vi "VMI_save_IF32_format.vi"(3 "Image Array":i16[][](array[numeric]), 4 "Image Info":T2={"X size"=782.0, "Y size"=582.0, "Centroiding"=1.0}, 5 "Header Cluster":T1) -> (2 "File String":string)   [LabVIEW 2018]
uses:
  Type defs/Image_info.ctl
  Type defs/Header_infor_IF32.ctl
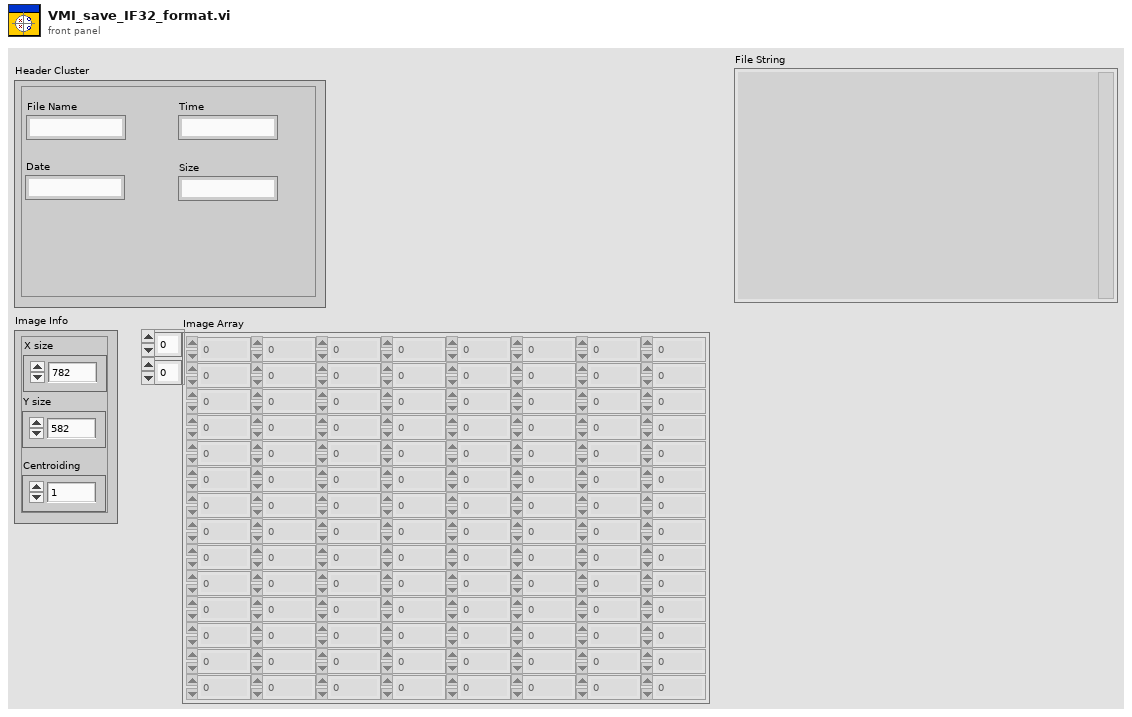
[diagram p1: front panel]
types:
  T1 = typedef "Header_infor_IF32.ctl" = cluster{"File Name":string, "Time":string, "Date":string, "Size":string}
  T2 = typedef "Image_info.ctl" = cluster{"X size":dbl, "Y size":dbl, "Centroiding":dbl}
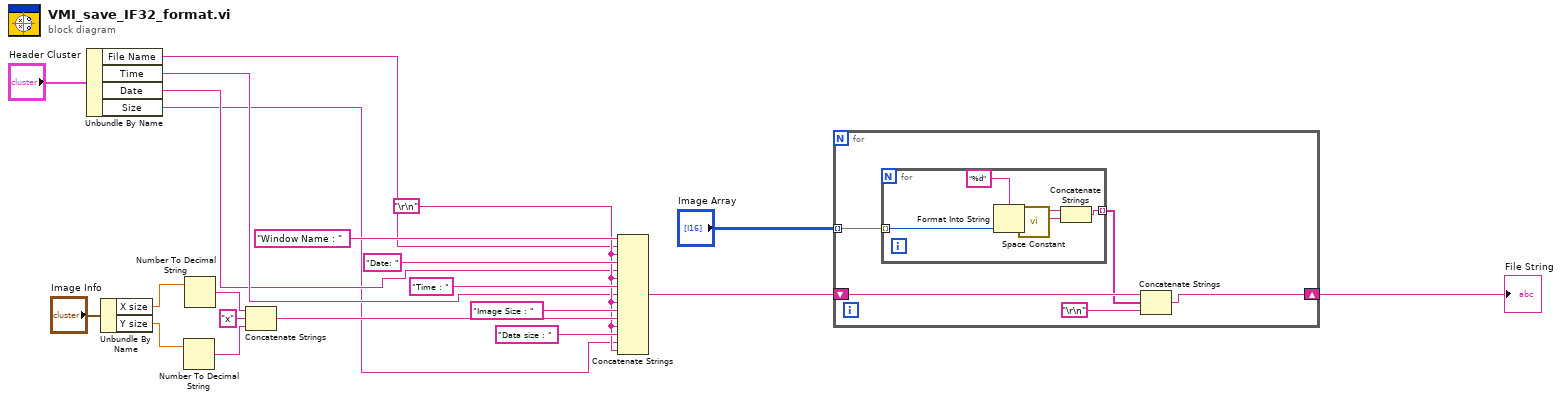
[diagram p0: block diagram]
diagram:
  w8 = "\r\n"
  n1 = Unbundle By Name("Header Cluster") -> ("File Name"=w4:string, "Time"=w3:string, "Date"=w2:string, "Size"=w1:string)
  n2 = Unbundle By Name("Image Info") -> ("X size"=w17:dbl, "Y size"=w16:dbl)
  n3 = Number To Decimal String(number=w16) -> (decimal integer string=w15:string)  [unwired: 1 in]
  n4 = Number To Decimal String(number=w17) -> (decimal integer string=w14:string)  [unwired: 1 in]
  n5 = Concatenate Strings(w14, "x" ("string"), w15) -> (w12:string)
  n6 = Concatenate Strings("Window Name : " ("string"), w4, w8, "Date: " ("string"), w2, w8, "Time : " ("string"), w3, w8, "Image Size : " ("string"), w12, w8, "Data size : " ("string"), w1, w8) -> (w7:string)
  n7 = for {
    tunnel: "Image Array" -> [w26] mode=indexing
    shift-right: [w22] -> w6
    shift-left: w7 -> [w25]
    n8 = for {
      tunnel: w26 -> [w31] mode=indexing
      tunnel: [w28] -> w24 mode=indexing
      n9 = Format Into String(format string="%d", w31) -> (resulting string=w30:string)  [unwired: 2 in, 1 out]
      n10 = call <vilib>:"Space Constant.vi"() -> ("String"=w27:string)
      n11 = Concatenate Strings(w30, w27) -> (w28:string)
    }
    n12 = Concatenate Strings(w25, w24, "\r\n") -> (w22:string)
  }
  "File String" <- w6
